vi "MultiPointConfigBroadcast.vi"(8 "error in (no error)":errorcluster, 10 "MultiPointConfig":T1 {"eSampleClock" items=["NULL"=0, "Immediate"=1, "External"=2, "Software Trigger"=3, "Interval"=10]}, 11 "ModuleID":i32) -> (0 "error out":errorcluster)   [LabVIEW 2014, in "SamplerPlugins.lvlib" / "SamplerPluginsBase.lvclass"]
uses:
  SamplerPluginsBase.lvclass
  TypeDefs/ConfigMultiPointParams.ctl
  SamplerModule/Protected/clEventType.ctl
  <vilib>/Utility/error.llb/Error Cluster From Error Code.vi
  <vilib>/ErrorRing/Error Ring.xnode
  SamplerModule/SamplerModule.lvlib
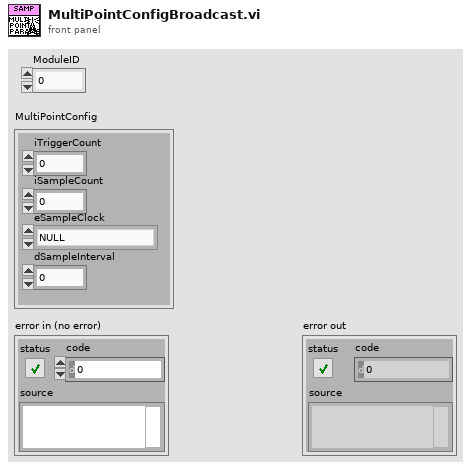
[diagram p1: front panel]
types:
  T1 = typedef "SamplerPlugins.lvlib/SamplerPluginsBase.lvclass/ConfigMultiPointParams.ctl" = cluster{"iTriggerCount":i32, "iSampleCount":i32, "eSampleClock":u16, "dSampleInterval":dbl}
  T2 = typedef "SamplerModule.lvlib/clBroadcastEvents.ctl" = cluster{"DidInit":refnum<user-event>, "StatusUpdate":refnum<user-event>, "ErrorReport":refnum<user-event>, "DidStop":refnum<user-event>, "PathToINI":refnum<user-event>, "GetReading":refnum<user-event>, "IsOverRange":refnum<user-event>, "GetMultiPointReading":refnum<user-event>, "MultiPointParams":refnum<user-event>, "MultiPointConfig":refnum<user-event>, "CorrFactors":refnum<user-event>}
  T3 = typedef "SamplerModule.lvlib/clEventType.ctl" = cluster{"ModuleID":i32, "Data":variant}
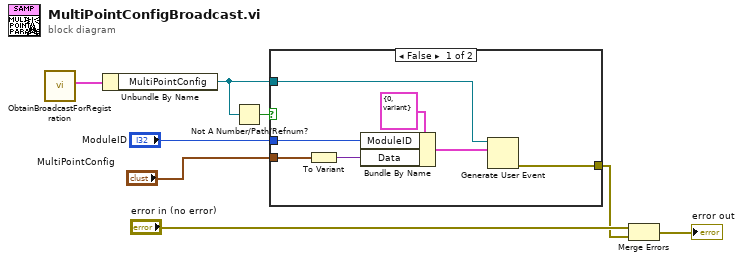
[diagram p0: block diagram]
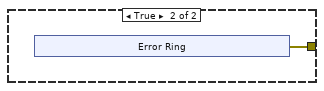
[diagram p2: hidden frame]
diagram:
  n1 = call "ObtainBroadcastForRegistration.vi"() -> ("SamplerBroadcast"=w8:T2)  [unwired: 10 in, 1 out]
  n2 = Unbundle By Name(w8) -> ("MultiPointConfig"=w3:refnum<user-event>)
  n3 = Not A Number/Path/Refnum?(number/path/refnum=w3) -> (NaN/Path/Refnum?=w4:bool)
  n4 = case shown="False" w4 {
    tunnel: "ModuleID" -> [w14 _]
    tunnel: "MultiPointConfig" -> [w12 _]
    tunnel: w3 -> [w10 _]
    tunnel: [w9 w16] -> w2
    frame False {
      n5 = To Variant(anything=w12) -> (Variant=w13:variant)
      n6 = Bundle By Name(cluster=T3 {"ModuleID"=0, "Data"=variant} ("clEventType"), "ModuleID"=w14, "Data"=w13) -> (w11:T3)
      n7 = Generate User Event(user event=w10, event data cluster=w11) -> (error out=w9:errorcluster)  [unwired: 2 in, 1 out]
    }
    frame True {
      n8 = xnode "Error Ring"() -> ("error out"=w16:errorcluster)
    }
  }
  n9 = Merge Errors("error in (no error)", w2) -> (→"error out":errorcluster)
